vi "XYZTheta Go.vi"(8 "error in (no error)":errorcluster, 10 "XYZTheta In":dbl[](array[numeric]), 11 "Gantry In":refnum<k24>) -> (0 "error out":errorcluster, 2 "XYZTheta Out":dbl[](array[numeric]), 3 "Gantry Out":refnum<k24>)   [LabVIEW 2019, in "A3200.lvclass"]
uses:
  A3200/A3200.lvclass
  C:/Program Files (x86)/Aerotech/A3200/LabVIEW/2010/Bin/Aerotech.A3200.dll
  Program Files (x86)/Aerotech/A3200/LabVIEW/2010/Bin/Aerotech.A3200.dll
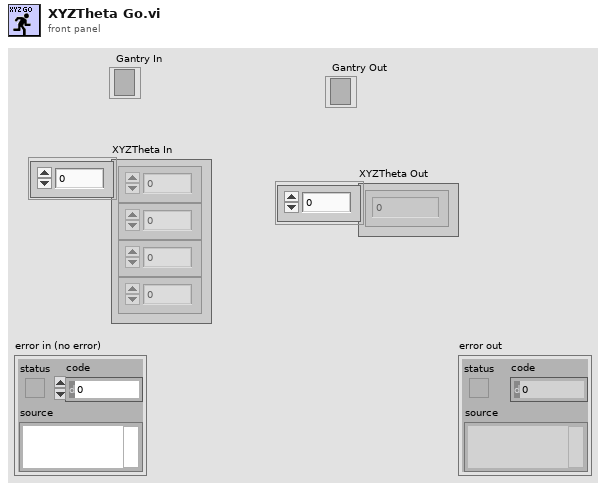
[diagram p1: front panel]
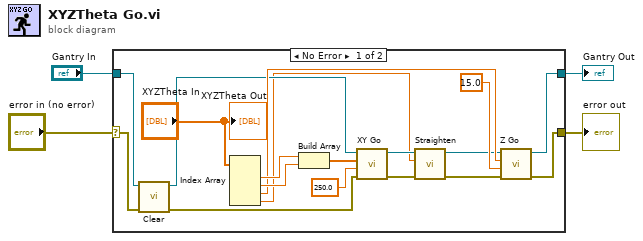
[diagram p0: block diagram]
diagram:
  n1 = case shown="No Error" "error in (no error)" {
    selector: "error in (no error)" -> [w9 w24]
    tunnel: [w5 w24] -> w3
    tunnel: "Gantry In" -> [w19 w23]
    tunnel: [w18 w23] -> w1
    frame No Error {
      n2 = call "Clear.vi"("error in (no error)"=w9, "Gantry In"=w19) -> ("error out"=w8:errorcluster, "Gantry Out"=w12:refnum<k24>)  [unwired: 8 in]
      n3 = Index Array(array="XYZTheta In") -> (element #1=w21:dbl, element #2=w22:dbl, element #3=w17:dbl, element #4=w10:dbl)  [unwired: 4 in]
      n4 = Build Array(w21, w22) -> (w13:dbl[])
      n5 = call "XY Go.vi"("error in (no error)"=w8, "Speed"=250.0, "XY"=w13, "Gantry In"=w12) -> ("error out"=w7:errorcluster, "Gantry Out"=w11:refnum<k24>)  [unwired: 6 in]
      n6 = call "Straighten.vi"("error in (no error)"=w7, "Angle (rad)"=w10, "Gantry In"=w11) -> ("error out"=w6:errorcluster, "Gantry Out"=w15:refnum<k24>)  [unwired: 7 in]
      n7 = call "Z Go.vi"("error in (no error)"=w6, "Speed"=15.0, "Position"=w17, "Gantry In"=w15) -> ("error out"=w5:errorcluster, "Gantry Out"=w18:refnum<k24>)  [unwired: 6 in]
      "XYZTheta Out" <- "XYZTheta In"
    }
    frame Error {
    }
  }
  "error out" <- w3
  "Gantry Out" <- w1
